vi "运行指示灯无信号处理.vi"(11 "ID 2":u32) -> (0 "4运行":bool, 1 "3运行":bool, 2 "2运行":bool, 3 "1运行":bool, 4 "5运行":bool)   [LabVIEW 2014]
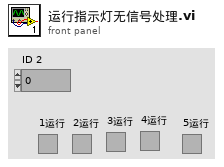
[diagram p1: front panel]
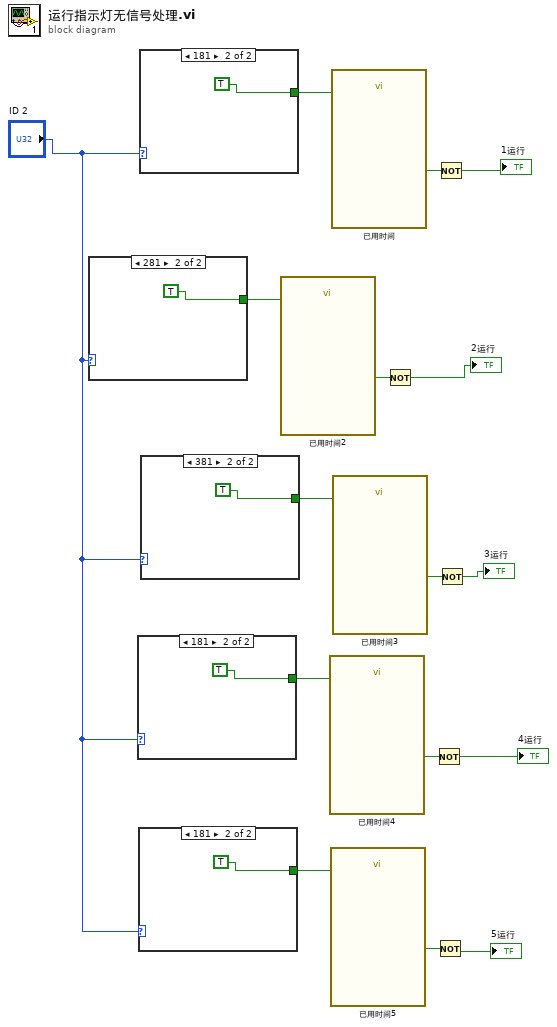
[diagram p0: block diagram]
diagram:
  n1 = case shown="281" "ID 2" {
    tunnel: [_ TRUE] -> w13
    frame 0, Default {
    }
    frame 641 {
    }
  }
  n2 = case shown="181" "ID 2" {
    tunnel: [_ TRUE] -> w7
    frame 0, Default {
    }
    frame 385 {
    }
  }
  n3 = case shown="181" "ID 2" {
    tunnel: [_ TRUE] -> w4
    frame 0, Default {
    }
    frame 385 {
    }
  }
  n4 = case shown="181" "ID 2" {
    tunnel: [_ TRUE] -> w16
    frame 0, Default {
    }
    frame 385 {
    }
  }
  n5 = case shown="381" "ID 2" {
    tunnel: [_ TRUE] -> w10
    frame 0, Default {
    }
    frame 897 {
    }
  }
  n6 = call "已用时间2"("Reset"=w13) -> ("Time has Elapsed"=w12:bool)  [unwired: 11 in, 7 out]
  n7 = call "已用时间4"("Reset"=w7) -> ("Time has Elapsed"=w6:bool)  [unwired: 11 in, 7 out]
  n8 = call "已用时间5"("Reset"=w4) -> ("Time has Elapsed"=w3:bool)  [unwired: 11 in, 7 out]
  n9 = call "已用时间"("Reset"=w16) -> ("Time has Elapsed"=w15:bool)  [unwired: 11 in, 7 out]
  n10 = call "已用时间3"("Reset"=w10) -> ("Time has Elapsed"=w9:bool)  [unwired: 11 in, 7 out]
  n11 = Not(x=w12) -> (.not. x?=→"2运行":bool)
  n12 = Not(x=w6) -> (.not. x?=→"4运行":bool)
  n13 = Not(x=w3) -> (.not. x?=→"5运行":bool)
  n14 = Not(x=w15) -> (.not. x?=→"1运行":bool)
  n15 = Not(x=w9) -> (.not. x?=→"3运行":bool)
